vi "数据截取保存.vi"(8 "错误输入（无错误）":errorcluster, 10 "TCP网络连接输入":refnum<k5>, 11 "read string":string="$50FBE0,FWD-1,E12,?,5657,?,?,2184,21,?,0.10,kgf.cm,400,0,GL1552,inner,100,A \r\n" caption="读取字符串") -> (0 "错误输出":errorcluster, 1 "CMD":string, 2 "连接ID输出":refnum<k5>, 3 "结果数组":string[](array[string]))   [LabVIEW 2011]
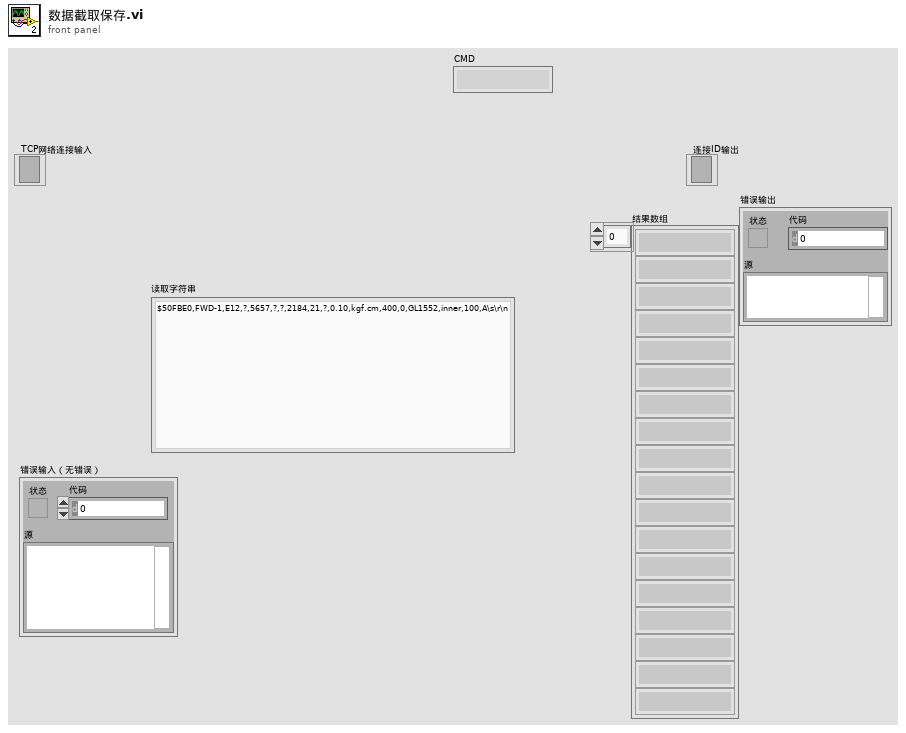
[diagram p1: front panel]
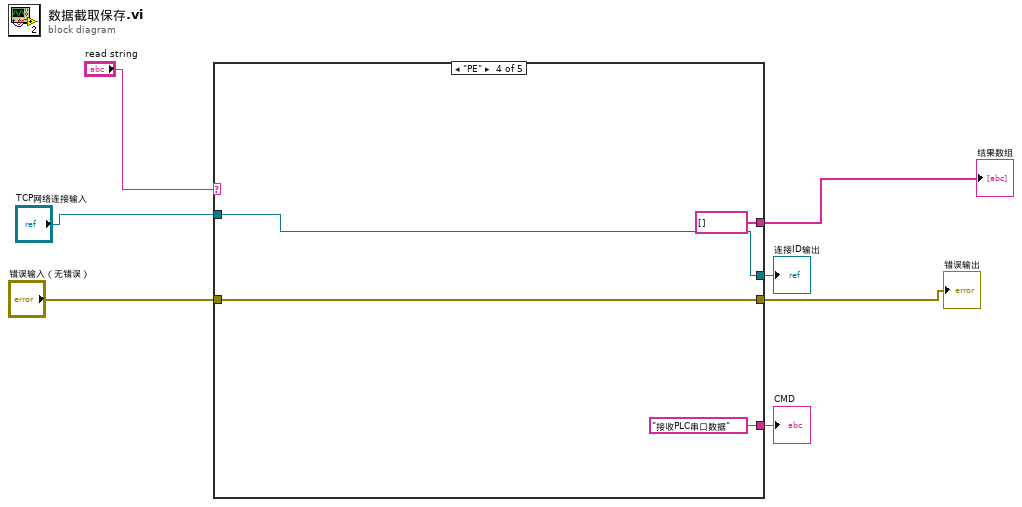
[diagram p0: block diagram]
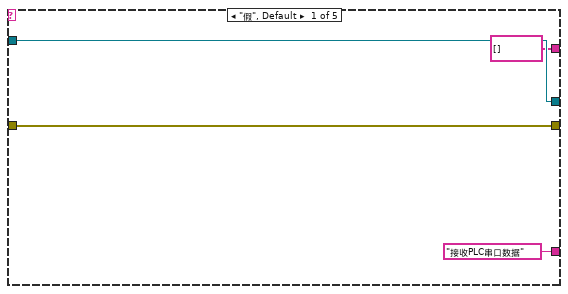
[diagram p2: hidden frame]
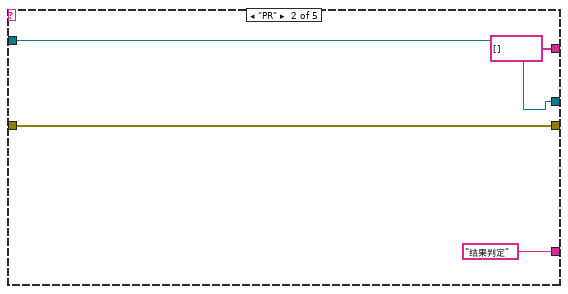
[diagram p3: hidden frame]
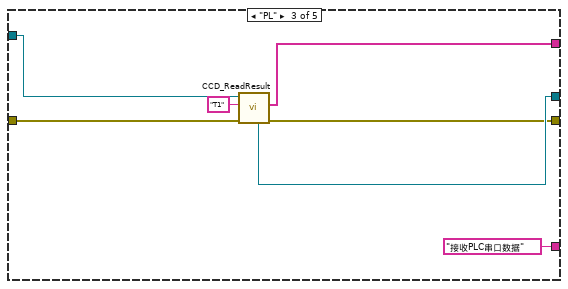
[diagram p4: hidden frame]
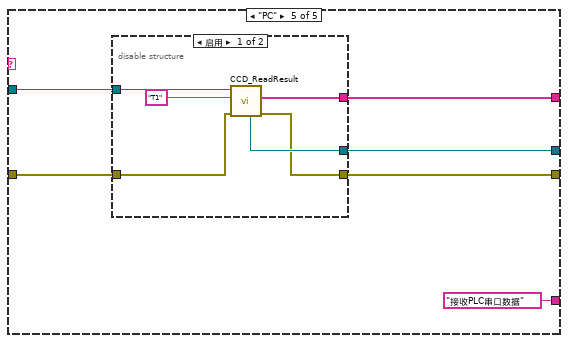
[diagram p5: hidden frame]
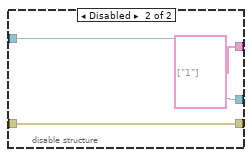
[diagram p6: hidden frame]
diagram:
  n1 = case shown="\"PE\"" "read string" {
    tunnel: "TCP网络连接输入" -> [w11 w15 w22 w26 w32]
    tunnel: [w11 w15 w21 w26 w31] -> w5
    tunnel: [string[] [] ("Array out") string[] [] ("Array out") w20 string[] [] ("Array out") w30] -> w4
    tunnel: "错误输入（无错误）" -> [w10 w14 w19 w25 w29]
    tunnel: [w10 w14 w18 w25 w28] -> w2
    tunnel: ["接收PLC串口数据" "结果判定" "接收PLC串口数据" "接收PLC串口数据" "接收PLC串口数据"] -> w1
    frame "假", Default {
    }
    frame "PR" {
    }
    frame "PL" {
      n2 = call "CCD_ReadResult.vi"("错误输入（无错误）"=w19, "Input Line"="T1", "TCP网络连接输入"=w22) -> ("错误输出"=w18:errorcluster, "Array out"=w20:string[], "连接ID输出"=w21:refnum<k5>)  [unwired: 3 in, 3 out]
    }
    frame "PE" {
    }
    frame "PC" {
      n3 = disable-structure shown="启用" {
        disable-tunnel: w32 -> [w38 w41]
        disable-tunnel: [w37 w41] -> w31
        disable-tunnel: [w36 string[] ["1"] ("Array out")] -> w30
        disable-tunnel: w29 -> [w35 w40]
        disable-tunnel: [w34 w40] -> w28
        frame Enabled {
          n4 = call "CCD_ReadResult.vi"("错误输入（无错误）"=w35, "Input Line"="T1" ("CMD:"), "TCP网络连接输入"=w38) -> ("错误输出"=w34:errorcluster, "Array out"=w36:string[], "连接ID输出"=w37:refnum<k5>)  [unwired: 3 in, 3 out]
        }
        frame Disabled {
        }
      }
    }
  }
  "结果数组" <- w4
  "连接ID输出" <- w5
  "错误输出" <- w2
  "CMD" <- w1
